vi "__setRoomItem.vi"(9 "room":T1, 10 "Room GUID":string, 11 "Room-API in":refnum<class "Room-API.lvclass">) -> (3 "Room-API out":refnum<class "Room-API.lvclass">)   [LabVIEW 2020, in "Room-API.lvclass"]
uses:
  Room-API.lvclass
  Single Room.ctl
  Room-API.lvclass/Room-API.ctl
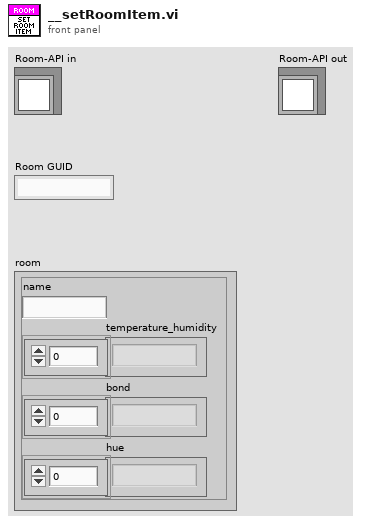
[diagram p1: front panel]
types:
  T1 = typedef "Room-API.lvclass/Single Room.ctl" = cluster{"name":string, "temperature_humidity":string[], "bond":string[], "hue":string[]}
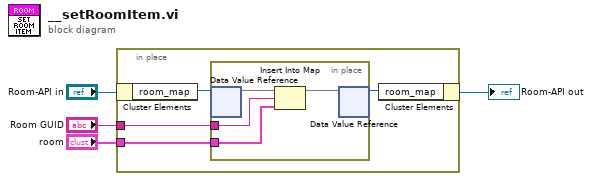
[diagram p0: block diagram]
diagram:
  n1 = in-place {
    in-place-border: "Room GUID" -> [w6]
    in-place-border: "room" -> [w5]
    n2 = in-place-cluster #1("Room-API in") -> ("room_map"=w8:refnum<data-value>)
    n3 = in-place {
      in-place-border: w6 -> [w10]
      in-place-border: w5 -> [w9]
      n4 = in-place-dvr #2(w8) -> (w12:map{string, T1})  [unwired: 1 out]
      n5 = Insert Into Map(map in=w12, key=w10, value=w9) -> (map out=w11:map{string, T1})  [unwired: 2 out]
      n6 = in-place-dvr #2(w11) -> (w7:refnum<data-value>)  [unwired: 1 out]
    }
    n7 = in-place-cluster #1("room_map"=w7) -> (→"Room-API out":refnum<class "Room-API.lvclass">)
  }
